vi "Teardown.vi"(8 "error in (no error)":errorcluster, 11 "1553 Unit Test in":refnum<class "Remote Terminal.lvclass">) -> (0 "error out":errorcluster)   [LabVIEW 2020, in "Unit Tests.lvlib" / "Remote Terminal.lvclass"]
uses:
  Remote Terminal.lvclass
  Utilities/Simulated FPGA/FPGA Sim.lvclass
  Remote Terminal.lvclass/Remote Terminal.ctl
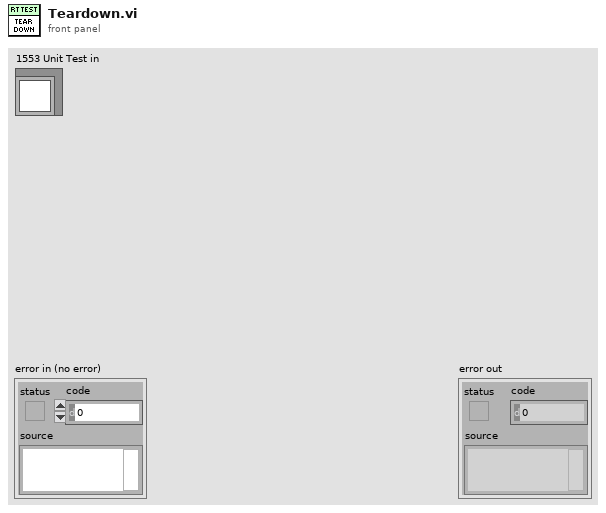
[diagram p1: front panel]
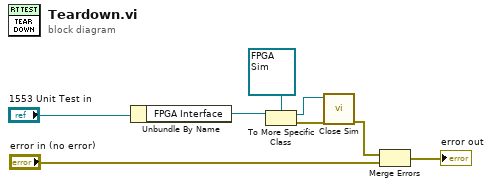
[diagram p0: block diagram]
diagram:
  n1 = Unbundle By Name("1553 Unit Test in") -> ("FPGA Interface"=w7:refnum<class "FPGA Interface.lvclass">)
  n2 = To More Specific Class(target class=refnum<class "FPGA Sim.lvclass"> refnum ("FPGA Sim.lvclass"), reference=w7) -> (specific class reference=w5:refnum<class "FPGA Sim.lvclass">, error out=w4:errorcluster)  [unwired: 1 in]
  n3 = call "Close Sim.vi"("error in (no error)"=w4, "FPGA Sim in"=w5) -> ("error out"=w3:errorcluster)  [unwired: 9 in]
  n4 = Merge Errors(w3, "error in (no error)") -> (→"error out":errorcluster)
